vi "Local to Global Point.vi"(10 "Car Info":T3, 11 "Local Point":T1) -> (3 "Global Point":T1)   [LabVIEW 2020, in "FormulaG-Common.lvlib"]
uses:
  FormulaG-Common.lvlib
  Point.ctl
  Coordinate Frame.ctl
  Car Info.ctl
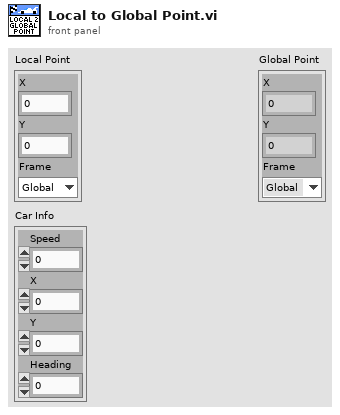
[diagram p1: front panel]
types:
  T1 = typedef "FormulaG-Common.lvlib/Point.ctl" = cluster{"X":sgl, "Y":sgl, "Frame":T2}
  T2 = typedef "FormulaG-Common.lvlib/Coordinate Frame.ctl" = enum16{"Global", "Local"}
  T3 = typedef "FormulaG-Common.lvlib/Car Info.ctl" = cluster{"Speed":sgl, "X":sgl, "Y":sgl, "Heading":sgl}
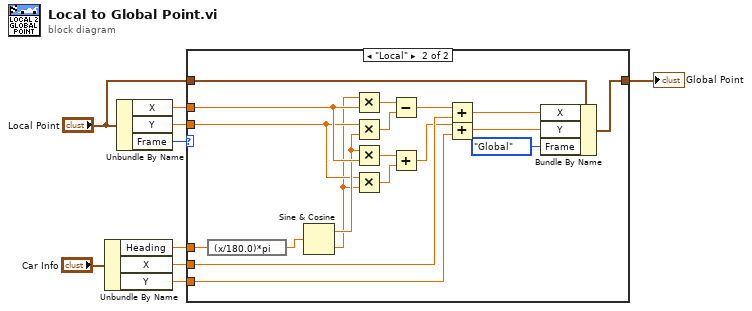
[diagram p0: block diagram]
diagram:
  n1 = Unbundle By Name("Car Info") -> ("Heading"=w8:sgl, "X"=w6:sgl, "Y"=w5:sgl)
  n2 = Unbundle By Name("Local Point") -> ("X"=w3:sgl, "Y"=w4:sgl, "Frame"=w7:T2)
  n3 = case shown="\"Local\"" w7 {
    tunnel: w8 -> [_ w29]
    tunnel: w6 -> [_ w23]
    tunnel: w5 -> [_ w22]
    tunnel: w4 -> [_ w13]
    tunnel: w3 -> [_ w15]
    tunnel: "Local Point" -> [w10 w28]
    tunnel: [w10 w26] -> w1
    frame "Global" {
    }
    frame "Local" {
      n4 = expression code="(x/180.0)*pi" ("degrees to radians")(w29) -> (w11:sgl)
      n5 = Sine & Cosine(0:w11) -> (1:w14:sgl, 2:w12:sgl)
      n6 = Multiply(x=w12, y=w15) -> (x*y=w21:sgl)
      n7 = Multiply(x=w13, y=w14) -> (x*y=w20:sgl)
      n8 = Multiply(x=w14, y=w15) -> (x*y=w17:sgl)
      n9 = Multiply(x=w13, y=w12) -> (x*y=w18:sgl)
      n10 = Subtract(x=w21, y=w20) -> (x-y=w19:sgl)
      n11 = Add(x=w17, y=w18) -> (x+y=w16:sgl)
      n12 = Add(x=w19, y=w23) -> (x+y=w25:sgl)
      n13 = Add(x=w16, y=w22) -> (x+y=w24:sgl)
      n14 = Bundle By Name(cluster=w28, "X"=w25, "Y"=w24, "Frame"=Coordinate_Frame."Global") -> (w26:T1)
    }
  }
  "Global Point" <- w1
